vi "MVC Starter.vi"() -> ()   [LabVIEW 2011]
doc: "This VI is a basic function generator."
uses:
  Controls/Command.ctl
  <vilib>/express/express analysis/Spectral/Block/exnSpectralBlock spectral measurements power poly.vi
  <vilib>/express/express analysis/Spectral/Block/exnSpectralBlock spectral measurements power WFM.vi
  <vilib>/express/express analysis/Spectral/XNode/ExpressSpectralMeasurementsBlockNode.xnode
panel:
  in  "FFT Signal":bool
  in  "Gen Signal":bool
  in  "Frequency":dbl(knob) scale=0.0..11.0
  out "Waveform Graph":waveform(dbl)(graph)
  in  "stop":bool
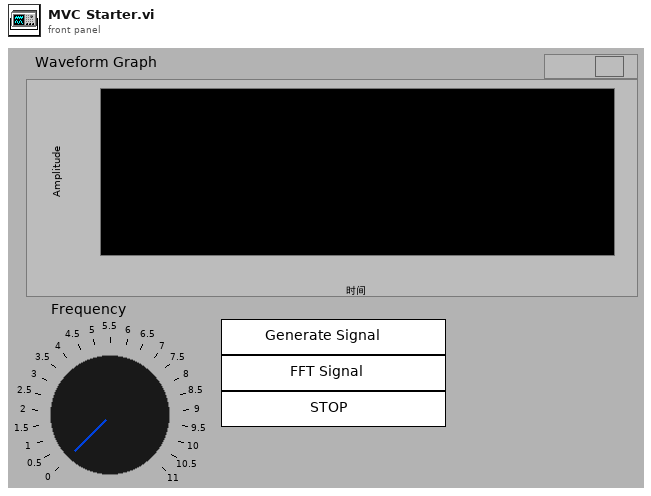
[diagram p1: front panel]
types:
  T1 = typedef "Command.ctl" = enum16{"Create Signal", "FFT Signal", "Set Frequency", "Stop", "Display", "Set Type"}
  T2 = cluster{"averaging mode":u16, "weighting mode":u16, "number of averages":u32}
  T3 = cluster{"dB On (F)":bool, "unwrap phase (F)":bool, "convert to degree (F)":bool}
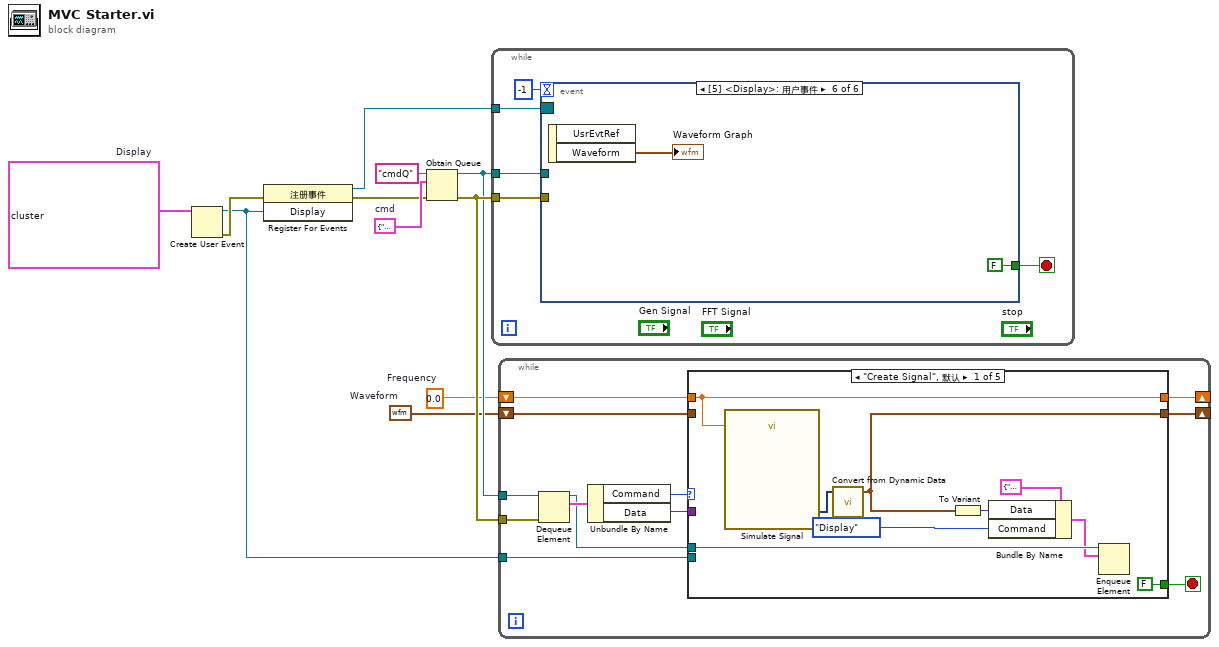
[diagram p0: block diagram]
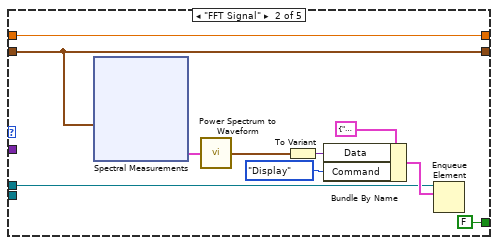
[diagram p2: hidden frame]
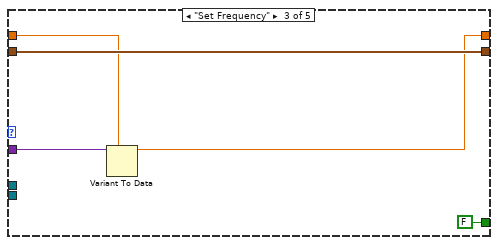
[diagram p3: hidden frame]
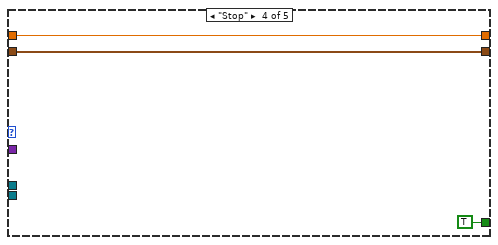
[diagram p4: hidden frame]
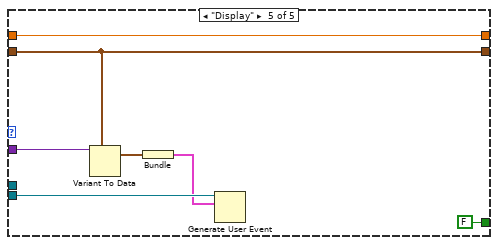
[diagram p5: hidden frame]
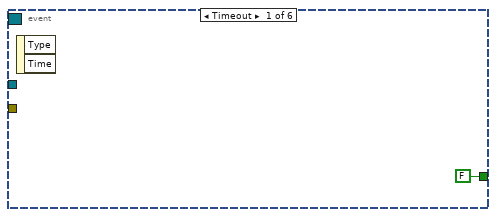
[diagram p6: hidden frame]
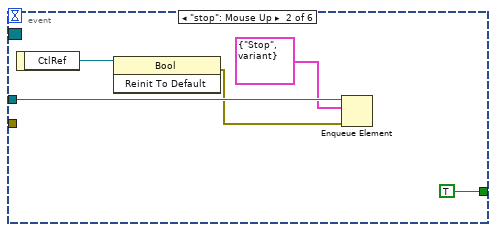
[diagram p7: hidden frame]
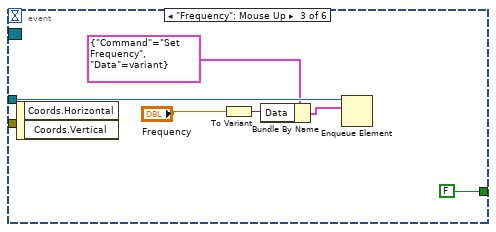
[diagram p8: hidden frame]
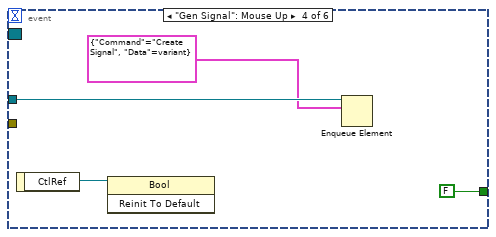
[diagram p9: hidden frame]
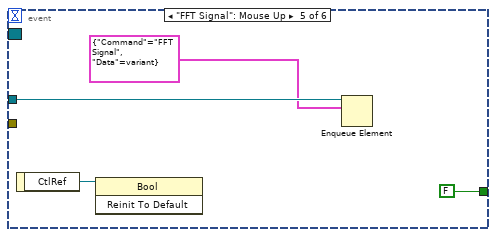
[diagram p10: hidden frame]
diagram:
  w2 = 0.0  # Frequency
  w3 = waveform(dbl) {"t0"=timestamp(0 s since 1904-01-01), "dt"=1.0, "Y"=[]}  # Waveform
  w8 = cluster{"Waveform":waveform(dbl)} {"Waveform"={"t0"=timestamp(0 s since 1904-01-01), "dt"=1.0, "Y"=[]}}  # Display
  w11 = cluster{"Command":T1, "Data":variant} {"Command"=enum."Create Signal", "Data"=variant}  # cmd
  n1 = Create User Event(user event datatype=w8) -> (user event=w1:refnum<user-event>, error out=w7:errorcluster)  [unwired: 1 in]
  n2 = register-events(error in=w7, w1) -> (reference out=w6:refnum<event-registration>, error out=w9:errorcluster)  [unwired: 1 in]
  n3 = Obtain Queue(name (unnamed)="cmdQ", element data type=w11, error in (no error)=w9) -> (queue out=w4:refnum<queue>, error out=w5:errorcluster)  [unwired: 2 in, 1 out]
  n4 = while {
    tunnel: w4 -> [w15]
    tunnel: w6 -> [w13]
    tunnel: w5 -> [w12]
    stop <- w14 stop-if-true
    n5 = event shown="[5] <Display>: 用户事件" {
      selector: w13 -> [_ _ _ _ _ _]
      dyn-events: _ -> [_ _ _ _ _ _]
      timeout: -1 -> [_ _ _ _ _ _]
      tunnel: w15 -> [_ w21 w28 w32 w36 _]
      tunnel: [FALSE TRUE FALSE FALSE FALSE FALSE] -> w14
      tunnel: w12 -> [_ _ _ _ _ _]
      event Timeout {
        n6 = event-data() -> ()  [unwired: 1 in, 2 out]
      }
      event "stop": Mouse Up {
        n7 = event-data() -> ("CtlRef"=w22:refnum<vi>)  [unwired: 1 in]
        n8 = invoke class="Bool" method="Reinit To Default"(reference=w22) -> (error out=w20:errorcluster)  [unwired: 2 in, 2 out]
        n9 = Enqueue Element(queue=w21, element=cluster{"Command":T1, "Data":variant} {"Command"=enum."Stop", "Data"=variant}, error in (no error)=w20) -> ()  [unwired: 1 in, 3 out]
      }
      event "Frequency": Mouse Up {
        n10 = event-data() -> ()  [unwired: 1 in, 2 out]
        n11 = To Variant(anything="Frequency") -> (Variant=w24:variant)
        n12 = Bundle By Name(cluster=cluster{"Command":T1, "Data":variant} {"Command"=enum."Set Frequency", "Data"=variant} ("element"), "Data"=w24) -> (w25:cluster{"Command":T1, "Data":variant})
        n13 = Enqueue Element(queue=w28, element=w25) -> ()  [unwired: 2 in, 3 out]
      }
      event "Gen Signal": Mouse Up {
        n14 = event-data() -> ("CtlRef"=w29:refnum<vi>)  [unwired: 1 in]
        n15 = invoke class="Bool" method="Reinit To Default"(reference=w29) -> ()  [unwired: 2 in, 3 out]
        n16 = Enqueue Element(queue=w32, element=cluster{"Command":T1, "Data":variant} {"Command"=enum."Create Signal", "Data"=variant}) -> ()  [unwired: 2 in, 3 out]
      }
      event "FFT Signal": Mouse Up {
        n17 = event-data() -> ("CtlRef"=w33:refnum<vi>)  [unwired: 1 in]
        n18 = invoke class="Bool" method="Reinit To Default"(reference=w33) -> ()  [unwired: 2 in, 3 out]
        n19 = Enqueue Element(queue=w36, element=cluster{"Command":T1, "Data":variant} {"Command"=enum."FFT Signal", "Data"=variant}) -> ()  [unwired: 2 in, 3 out]
      }
      event User Event {
        n20 = event-data() -> ("Waveform"=→"Waveform Graph":waveform(dbl))  [unwired: 1 in, 1 out]
      }
    }
  }
  n21 = while {
    tunnel: w5 -> [w49]
    tunnel: w4 -> [w50]
    shift-right: [w43] -> _
    shift-left: w3 -> [w44]
    shift-right: [w40] -> _
    shift-left: w2 -> [w42]
    tunnel: w1 -> [w39]
    stop <- w45 stop-if-true
    n22 = Dequeue Element(queue=w50, error in (no error)=w49) -> (queue out=w41:refnum<queue>, element=w48:cluster{"Command":T1, "Data":variant})  [unwired: 1 in, 2 out]
    n23 = Unbundle By Name(w48) -> ("Command"=w47:T1, "Data"=w46:variant)
    n24 = case shown="\"Create Signal\", 默认" w47 {
      tunnel: w46 -> [_ _ w82 _ w91]
      tunnel: [FALSE FALSE FALSE TRUE FALSE] -> w45
      tunnel: w44 -> [_ w62 w83 w84 w90]
      tunnel: [w55 w62 w83 w84 w90] -> w43
      tunnel: w42 -> [w51 w69 w81 w86 w93]
      tunnel: w41 -> [w58 w64 _ _ _]
      tunnel: [w51 w69 w80 w86 w93] -> w40
      tunnel: w39 -> [_ _ _ _ w92]
      frame "Create Signal", Default {
        n25 = call "Simulate Signal"("Frequency"=w51) -> ("Sine"=w59:dynamicdata)  [unwired: 13 in, 1 out]
        n26 = call "Convert from Dynamic Data"("Dynamic Data Type"=w59) -> ("Waveform"=w55:waveform(dbl))  [unwired: 3 in]
        n27 = To Variant(anything=w55) -> (Variant=w54:variant)
        n28 = Bundle By Name(cluster=cluster{"Command":T1, "Data":variant} {"Command"=enum."Create Signal", "Data"=variant} ("element"), "Data"=w54, "Command"=Command."Display") -> (w53:cluster{"Command":T1, "Data":variant})
        n29 = Enqueue Element(queue=w58, element=w53) -> ()  [unwired: 2 in, 3 out]
      }
      frame "FFT Signal" {
        n30 = xnode "Spectral Measurements"("信号"=w62) -> ("Power Spectrum"=w61:cluster{"f0":dbl, "df":dbl, "magnitude":dbl[]})  [unwired: 1 in, 1 out]
        n31 = call "Power Spectrum to Waveform.vi"("Power Spectrum"=w61) -> ("Waveform"=w60:waveform(dbl))
        n32 = To Variant(anything=w60) -> (Variant=w66:variant)
        n33 = Bundle By Name(cluster=cluster{"Command":T1, "Data":variant} {"Command"=enum."Create Signal", "Data"=variant} ("element"), "Data"=w66, "Command"=Command."Display") -> (w65:cluster{"Command":T1, "Data":variant})
        n34 = Enqueue Element(queue=w64, element=w65) -> ()  [unwired: 2 in, 3 out]
      }
      frame "Set Frequency" {
        n35 = Variant To Data(type=w81, Variant=w82) -> (data=w80:dbl)  [unwired: 1 in, 1 out]
      }
      frame "Stop" {
      }
      frame "Display" {
        n36 = Variant To Data(type=w90, Variant=w91) -> (data=w89:waveform(dbl))  [unwired: 1 in, 1 out]
        n37 = Bundle("Waveform"=w89) -> (w88:cluster{"Waveform":waveform(dbl)})  [unwired: 1 in]
        n38 = Generate User Event(user event=w92, event data cluster=w88) -> ()  [unwired: 1 in, 2 out]
      }
    }
  }
